vi "Configure IF Ranging Port.vi"(8 "error in (no error)":errorcluster, 10 "Ranging IF Port Mode (0: Fast)":u16(ring) items=["Fast", "Normal"], 11 "VISA resource name":refnum<visa-resource-name>) -> (0 "error out":errorcluster, 3 "VISA resource name out":refnum<visa-resource-name>)   [LabVIEW 2020, in "Agilent ENA Series.lvlib"]
doc: "Sets the mode for the IF Ranging port.\n\nNote:\nValid for E5072A only"
uses:
  <instrlib>/Agilent ENA Series/Agilent ENA Series.lvlib
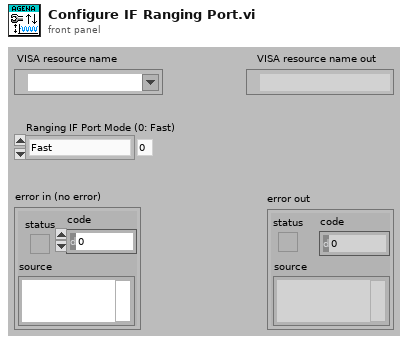
[diagram p1: front panel]
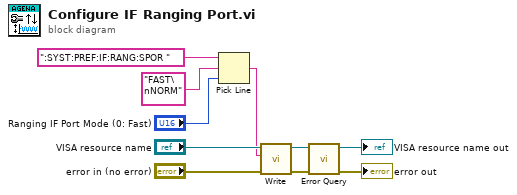
[diagram p0: block diagram]
diagram:
  n1 = Pick Line(string ("")=":SYST:PREF:IF:RANG:SPOR " ("format string"), multi-line string="FAST\nNORM", line index="Ranging IF Port Mode (0: Fast)") -> (output string=w1:string)
  n2 = call <instrlib>:"Write.vi"("error in (no error)"="error in (no error)", "String ()"=w1, "VISA resource name"="VISA resource name") -> ("error out"=w8:errorcluster, "VISA resource name out"=w7:refnum<visa-resource-name>)  [unwired: 6 in, 1 out]
  n3 = call <instrlib>:"Error Query.vi"("error in (no error)"=w8, "VISA resource name"=w7) -> ("error out"=→"error out":errorcluster, "VISA resource name out"=→"VISA resource name out":refnum<visa-resource-name>)  [unwired: 6 in, 2 out]
